vi "Derivative Control Points.vi"(11 "ctrl points":cluster{dbl, dbl}[](array[cluster])) -> (3 "d ctrl pts":cluster{dbl, dbl}[](array[cluster]))   [LabVIEW 2019]
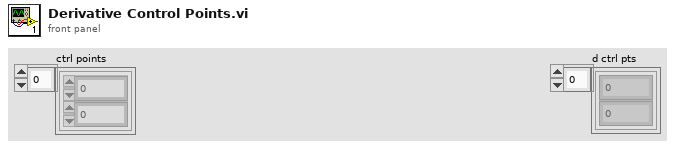
[diagram p1: front panel]
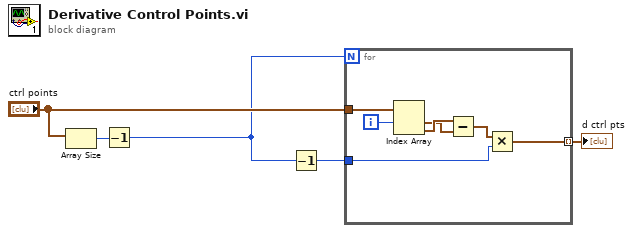
[diagram p0: block diagram]
diagram:
  n1 = Array Size(array="ctrl points") -> (size(s)=w5:i32)
  n2 = Decrement(x=w5) -> (x-1=w3:i32)
  n3 = Decrement(x=w3) -> (x-1=w2:i32)
  n4 = for {
    N: w3 -> [_]
    tunnel: "ctrl points" -> [w12]
    tunnel: w2 -> [w7]
    tunnel: [w6] -> w1 mode=indexing
    i -> [w11]
    n5 = Index Array(array=w12, index #1=w11) -> (element #1=w9:cluster{dbl, dbl}, element #2=w10:cluster{dbl, dbl})  [unwired: 1 in]
    n6 = Subtract(x=w10, y=w9) -> (x-y=w8:cluster{dbl, dbl})
    n7 = Multiply(x=w8, y=w7) -> (x*y=w6:cluster{dbl, dbl})
  }
  "d ctrl pts" <- w1
